vi "SVA 4MV6 T013 CCEl.vi"(9 "B":u8(slide) scale=0.0..255.0, 10 "G":u8(slide) scale=0.0..255.0, 11 "R":u8(slide) scale=0.0..255.0) -> (1 "V":dbl(slide) scale=0.0..1.0, 2 "S":dbl(slide) scale=0.0..1.0, 3 "H":dbl(knob))   [LabVIEW 2020]
doc: "Este vi realiza la conversion de un valor del sistema RGB (0 a 255) a HVS (0 a 1)"
panel:
  out "Color":u32(colorbox)
  # "Ceballos Conde Emanuel"
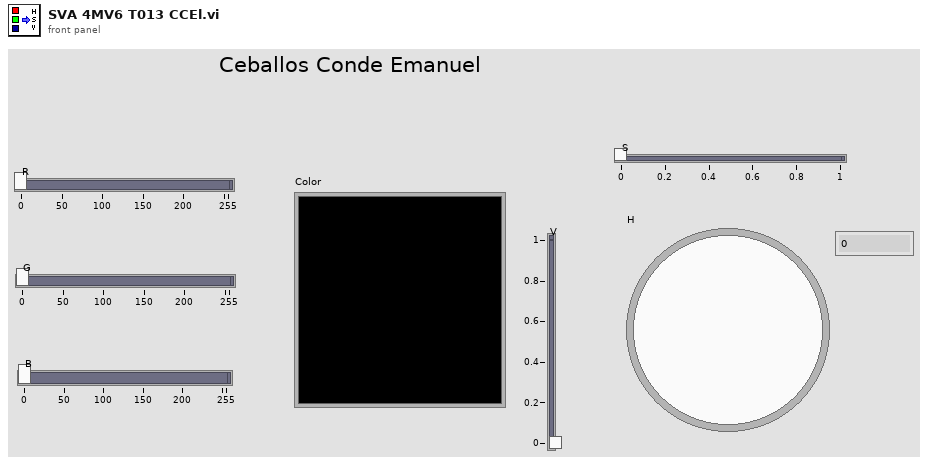
[diagram p1: front panel]
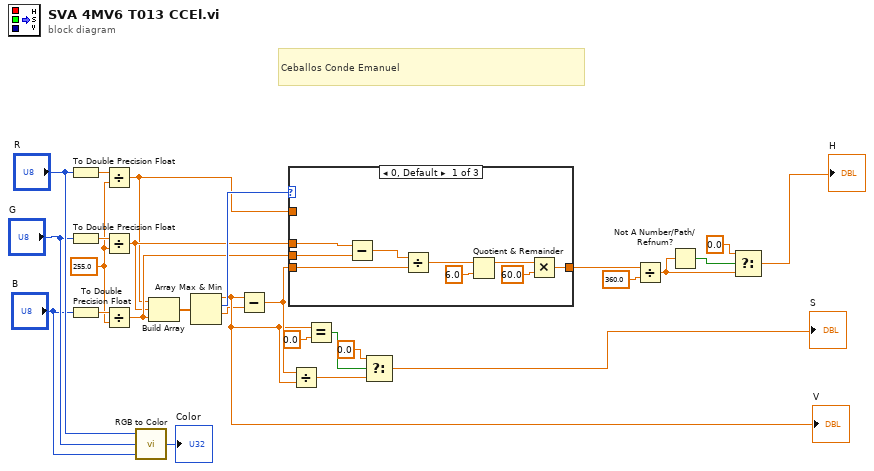
[diagram p0: block diagram]
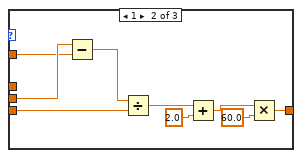
[diagram p2: hidden frame]
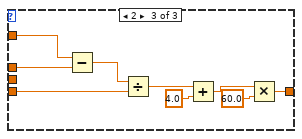
[diagram p3: hidden frame]
diagram:
  w5 = 255.0 ("y")
  # "Ceballos Conde Emanuel"
  n1 = To Double Precision Float(number="R") -> (double precision float=w6:dbl)
  n2 = To Double Precision Float(number="G") -> (double precision float=w7:dbl)
  n3 = To Double Precision Float(number="B") -> (double precision float=w8:dbl)
  n4 = Divide(x=w6, y=w5) -> (x/y=w20:dbl)
  n5 = Divide(x=w7, y=w5) -> (x/y=w21:dbl)
  n6 = Divide(x=w8, y=w5) -> (x/y=w22:dbl)
  n7 = call <vilib>:"RGB to Color.vi"("B"="B", "G"="G", "R"="R") -> ("Color"=→"Color":u32)
  n8 = Build Array(w20, w21, w22) -> (w9:dbl[])
  n9 = Array Max & Min(array=w9) -> (max value=w15:dbl, max index (indices)=w27:i32, min value=w13:dbl)  [unwired: 1 out]
  "V" <- w15
  n10 = Subtract(x=w15, y=w13) -> (x-y=w17:dbl)
  n11 = case shown="0, Default" w27 {
    tunnel: [w30 w39 w48] -> w18
    tunnel: w21 -> [w29 _ w46]
    tunnel: w22 -> [w28 w38 _]
    tunnel: w17 -> [w35 w44 w53]
    tunnel: w20 -> [_ w37 w47]
    frame 0, Default {
      n12 = Subtract(x=w29, y=w28) -> (x-y=w36:dbl)
      n13 = Divide(x=w36, y=w35) -> (x/y=w34:dbl)
      n14 = Quotient & Remainder(x=w34, y=6.0) -> (x-y*floor(x/y)=w31:dbl)  [unwired: 1 out]
      n15 = Multiply(x=w31, y=60.0) -> (x*y=w30:dbl)
    }
    frame 1 {
      n16 = Subtract(x=w38, y=w37) -> (x-y=w45:dbl)
      n17 = Divide(x=w45, y=w44) -> (x/y=w43:dbl)
      n18 = Add(x=w43, y=2.0) -> (x+y=w40:dbl)
      n19 = Multiply(x=w40, y=60.0) -> (x*y=w39:dbl)
    }
    frame 2 {
      n20 = Subtract(x=w47, y=w46) -> (x-y=w54:dbl)
      n21 = Divide(x=w54, y=w53) -> (x/y=w52:dbl)
      n22 = Add(x=w52, y=4.0) -> (x+y=w49:dbl)
      n23 = Multiply(x=w49, y=60.0) -> (x*y=w48:dbl)
    }
  }
  n24 = Divide(x=w17, y=w15) -> (x/y=w14:dbl)
  n25 = Equal?(x=w15, y=0.0) -> (x = y?=w11:bool)
  n26 = Select(t=0.0, s=w11, f=w14) -> (s? t:f=→"S":dbl)
  n27 = Divide(x=w18, y=360.0) -> (x/y=w24:dbl)
  n28 = Not A Number/Path/Refnum?(number/path/refnum=w24) -> (NaN/Path/Refnum?=w23:bool)
  n29 = Select(t=0.0, s=w23, f=w24) -> (s? t:f=→"H":dbl)
